vi "CalibrationStart.vi"(11 "Booléen":bool) -> ()   [LabVIEW 2020]
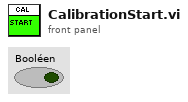
[diagram p1: front panel]
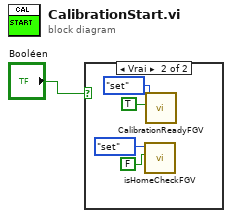
[diagram p0: block diagram]
diagram:
  n1 = case shown="Vrai" "Booléen" {
    frame False {
    }
    frame True {
      n2 = call "isHomeCheckFGV.vi"("isHomeCheck?"=FALSE, "state"=enum16{"get", "set"}."set") -> ()  [unwired: 9 in, 1 out]
      n3 = call "CalibrationReadyFGV.vi"("Énum"=enum16{"get", "1stClk", "set"}."set", "set"=TRUE) -> ()  [unwired: 8 in, 1 out]
    }
  }
